vi "Test List.vi"() -> ()   [LabVIEW 2014, in "FTP.lvlib" / "FTP.lvclass"]
uses:
  FTP.lvclass
panel:
  out "Raw List as String":string
  out "Error Out":errorcluster
  in  "passWord":string
  in  "userName":string
  in  "address":string
  out "Status":string
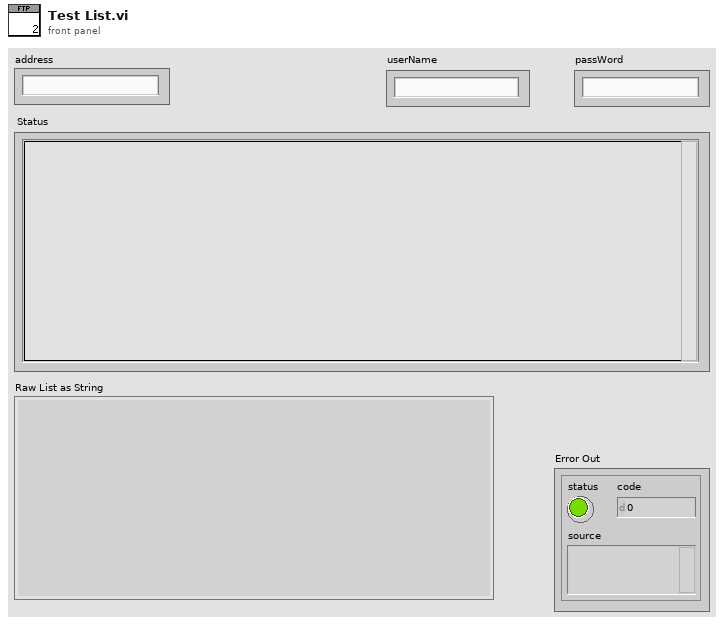
[diagram p1: front panel]
types:
  T1 = typedef "FTP.lvclass/CmdCluster.ctl" = cluster{"CmdSting":string, "FromClient":bool}
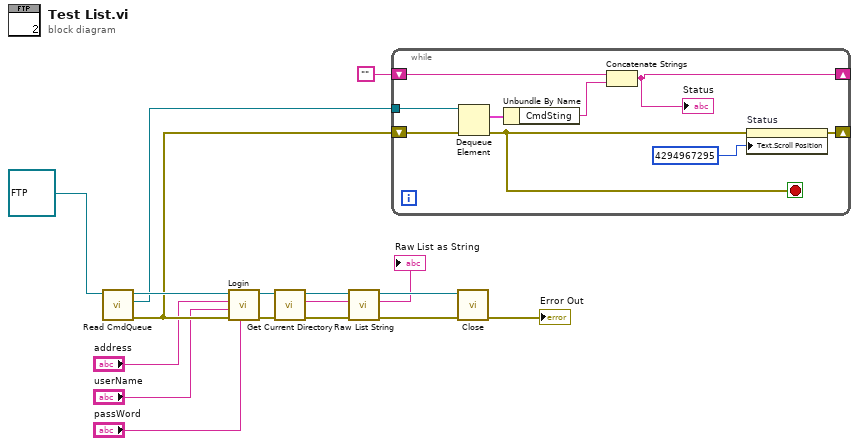
[diagram p0: block diagram]
diagram:
  n1 = call "Read CmdQueue.vi"("FTP in"=refnum<class "FTP.lvclass"> refnum) -> ("error out"=w8:errorcluster, "CmdQueue"=w9:refnum<queue>, "FTP out"=w17:refnum<class "FTP.lvclass">)  [unwired: 8 in]
  n2 = call "Login.vi"("passWord"="passWord", "error in (no error)"=w8, "userName"="userName", "address"="address", "FTP in"=w17) -> ("error out"=w1:errorcluster, "FTP out"=w2:refnum<class "FTP.lvclass">)  [unwired: 5 in]
  n3 = call "Get Current Directory.vi"("error in (no error)"=w1, "FTP in"=w2) -> ("error out"=w16:errorcluster, "Current Directory"=w12:string, "FTP out"=w15:refnum<class "FTP.lvclass">)  [unwired: 7 in]
  n4 = call "Raw List String.vi"("error in (no error)"=w16, "Remote File"=w12, "FTP in"=w15) -> ("error out"=w13:errorcluster, "Raw List as String"=→"Raw List as String":string, "FTP out"=w14:refnum<class "FTP.lvclass">)  [unwired: 6 in]
  n5 = while {
    tunnel: w9 -> [w26]
    shift-right: [w20] -> _
    shift-left: w8 -> [w25]
    shift-right: [w21] -> _
    shift-left: "" -> [w23]
    stop <- w18 stop-if-true
    n6 = Dequeue Element(queue=w26, error in (no error)=w25) -> (element=w24:T1, error out=w18:errorcluster)  [unwired: 1 in, 2 out]
    n7 = Unbundle By Name(w24) -> ("CmdSting"=w22:string)
    n8 = Concatenate Strings(w23, w22) -> (w21:string)
    "Status" <- w21
    n9 = property on="Status" class="Str"(error in=w18, "Text.Scroll Position"=u32 4294967295) -> (error out=w20:errorcluster)  [unwired: 1 in, 1 out]
  }
  n10 = call "Close.vi"("error in (no error)"=w13, "FTP in"=w14) -> ("error out"=→"Error Out":errorcluster)  [unwired: 9 in]
